vi "Run Auto Score.vi"(11 "Zip":path) -> (3 "Result":T1)   [LabVIEW 2024, in "Word Search Scorer.lvlib"]
uses:
  Word Search Scorer.lvlib
  Scoring Result.ctl
  <vilib>/Utility/error.llb/DialogType.ctl
  Result.ctl
  b176729e-45e3-4042-bf0b-439ceafae7e1.vi
  10f0845f-5e3d-49fd-8ad4-61868670d3b0.vi
panel:
  out "#":i32
  out "Additional Runs":i32
  out "Initial Run Time":dbl format="%_6f"
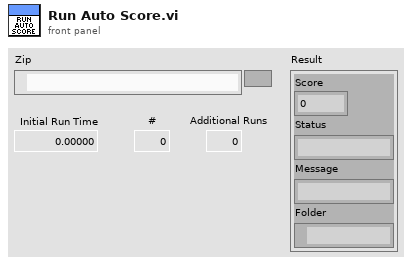
[diagram p1: front panel]
types:
  T1 = typedef "Word Search Scorer.lvlib/Scoring Result.ctl" = cluster{"Score":dbl, "Status":string, "Message":string, "Folder":path}
  T2 = typedef "DialogType.ctl" = u16
  T3 = typedef "Word Search Scorer.lvlib/Result.ctl" = enum16{"failed", "complete", "error", "timeout", "ineligible"}
  T4 = typedef "Word Search Scorer.lvlib/Solver VI Ref Type.ctl" = refnum<vi>
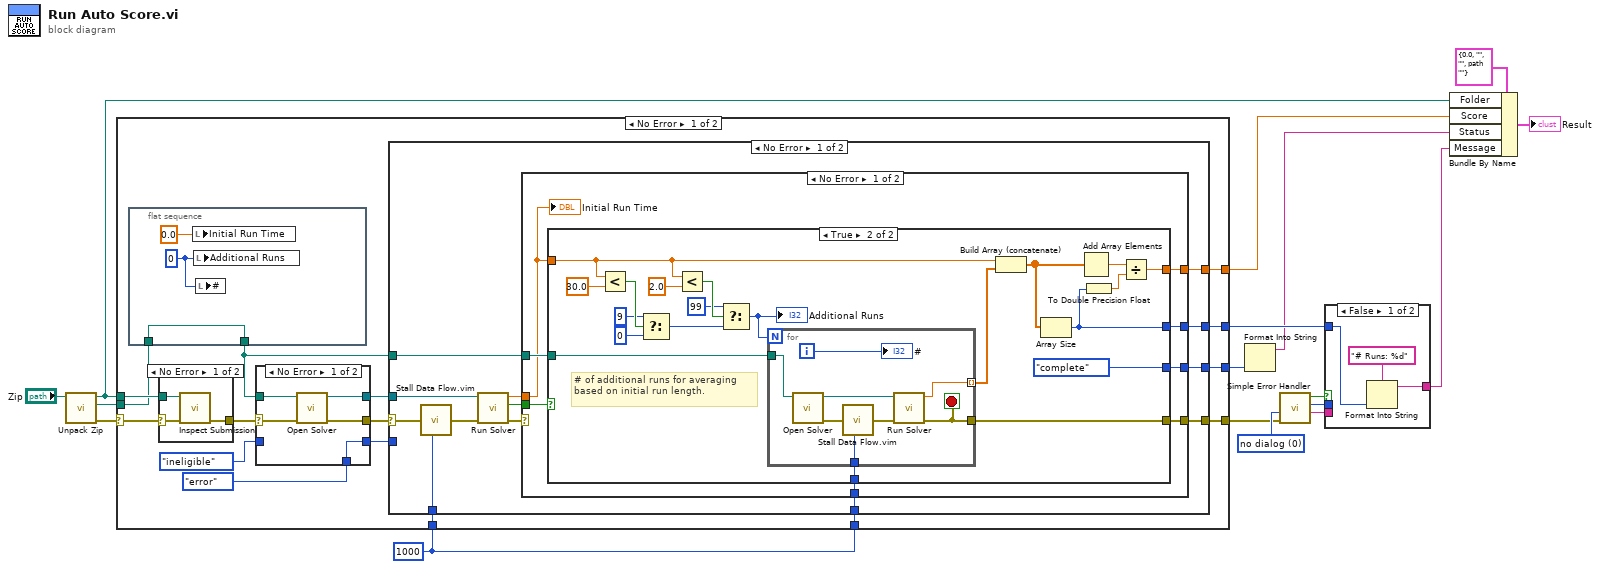
[diagram p0: block diagram]
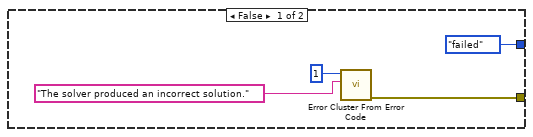
[diagram p2: hidden frame]
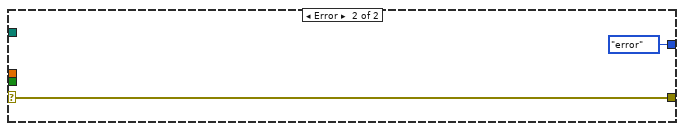
[diagram p3: hidden frame]
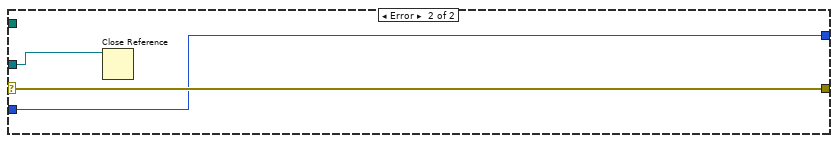
[diagram p4: hidden frame]
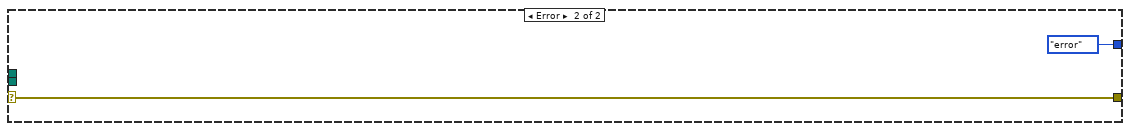
[diagram p7: hidden frame]
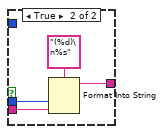
[diagram p8: hidden frame]
diagram:
  w1 = u32 1000 ("milliseconds to wait")
  w9 = T2 0 items=["no dialog", "OK message", "continue or stop message", "OK message + warnings", "continue/stop + warnings"] ("type of dialog (OK msg:1)")
  n1 = call "Unpack Zip.vi"("Zip"="Zip") -> ("error out"=w16:errorcluster, "Solver VI"=w13:path, "Folder"=w4:path)  [unwired: 8 in]
  n2 = case shown="No Error" w16 {
    selector: w16 -> [w33 w106]
    tunnel: w4 -> [w29 _]
    tunnel: w13 -> [w20 _]
    tunnel: [w25 Result."error" ("Result")] -> w8
    tunnel: [w24 w106] -> w7
    tunnel: [w23 _] -> w6
    tunnel: [w22 _] -> w5
    tunnel: w1 -> [w19 _]
    tunnel: w1 -> [w18 _]
    frame No Error {
      n3 = flat-sequence {
        tunnel: [w36] -> w21
        tunnel: w20 -> [w36]
        frame #0 {
          w34 = 0 ("Additional Runs")
          n4 = local write "Initial Run Time"(0.0 ("Initial Run Time")) -> ()
          n5 = local write "Additional Runs"(w34) -> ()
          n6 = local write "#"(w34) -> ()
        }
      }
      n7 = case shown="No Error" w33 {
        selector: w33 -> [w103 w105]
        tunnel: w29 -> [w104 _]
        tunnel: [w102 w105] -> w32
        frame No Error {
          n8 = call "Inspect Submission.vi"("error in (no error)"=w103, "Folder"=w104) -> ("error out"=w102:errorcluster)  [unwired: 7 in, 2 out]
        }
        frame Error {
        }
      }
      n9 = case shown="No Error" w32 {
        selector: w32 -> [w98 w101]
        tunnel: w21 -> [w99 _]
        tunnel: [w97 _] -> w30
        tunnel: [w96 w101] -> w31
        tunnel: [w95 w100] -> w27
        tunnel: Result."error" ("Result") -> [w95 _]
        tunnel: Result."ineligible" ("Result") -> [_ w100]
        frame No Error {
          n10 = call "Open Solver.vi"("error in (no error)"=w98, "Solver Path"=w99) -> ("error IO"=w96:errorcluster, "Solver VI"=w97:T4)  [unwired: 8 in]
        }
        frame Error {
        }
      }
      n11 = case shown="No Error" w31 {
        selector: w31 -> [w48 w94]
        tunnel: w30 -> [w49 w93]
        tunnel: [w43 w94] -> w24
        tunnel: w21 -> [w44 _]
        tunnel: [w42 _] -> w22
        tunnel: [w41 w92] -> w25
        tunnel: [w40 _] -> w23
        tunnel: w27 -> [_ w92]
        tunnel: w19 -> [w38 _]
        tunnel: w18 -> [w37 _]
        frame No Error {
          n12 = call "Stall Data Flow.vim"("value in"=w48, "milliseconds to wait"=w38) -> ("value out"=w39:errorcluster)  [unwired: 1 out]
          n13 = call "Run Solver.vi"("error in (no error)"=w39, "Solver VI"=w49) -> ("error out"=w47:errorcluster, "Completed"=w46:bool, "Run Time"=w45:dbl)  [unwired: 7 in]
          n14 = case shown="No Error" w47 {
            selector: w47 -> [_ w91]
            tunnel: w46 -> [w57 _]
            tunnel: w45 -> [w51 _]
            tunnel: w44 -> [w56 _]
            tunnel: [w55 w91] -> w43
            tunnel: [w54 _] -> w42
            tunnel: [w53 Result."error" ("Result")] -> w41
            tunnel: [w52 _] -> w40
            tunnel: w37 -> [w50 _]
            frame No Error {
              n15 = case shown="True" w57 {
                tunnel: w51 -> [_ w71]
                tunnel: w56 -> [_ w73]
                tunnel: [w60 w72] -> w55
                tunnel: [_ w66] -> w54
                tunnel: [Result."failed" ("Result") Result."complete" ("Result")] -> w53
                tunnel: [_ w64] -> w52
                tunnel: w50 -> [_ w62]
                frame False {
                  n16 = call <vilib>:"Error Cluster From Error Code.vi"("error message (\"\")"="The solver produced an incorrect solution.", "error code (0)"=1) -> ("error out"=w60:errorcluster)  [unwired: 7 in]
                }
                frame True {
                  # "# of additional runs for averaging based on initial run length."
                  n17 = Less?(x=w71, y=30.0) -> (x < y?=w80:bool)
                  n18 = Select(t=9, s=w80, f=0) -> (s? t:f=w76:i32)
                  n19 = Less?(x=w71, y=2.0) -> (x < y?=w75:bool)
                  n20 = Select(t=99, s=w75, f=w76) -> (s? t:f=w63:i32)
                  "Additional Runs" <- w63
                  n21 = for {
                    N: w63 -> [_]
                    tunnel: w73 -> [w87]
                    tunnel: [w86] -> w72
                    tunnel: [w85] -> w70 mode=indexing
                    tunnel: w62 -> [w82]
                    i -> [w84]
                    stop <- w86 stop-if-true
                    n22 = call "Open Solver.vi"("Solver Path"=w87) -> ("error IO"=w88:errorcluster, "Solver VI"=w89:T4)  [unwired: 9 in]
                    n23 = call "Stall Data Flow.vim"("value in"=w88, "milliseconds to wait"=w82) -> ("value out"=w83:errorcluster)  [unwired: 1 out]
                    n24 = call "Run Solver.vi"("error in (no error)"=w83, "Solver VI"=w89) -> ("error out"=w86:errorcluster, "Run Time"=w85:dbl)  [unwired: 7 in, 1 out]
                    "#" <- w84
                  }
                  n25 = Build Array (concatenate)(w71, w70) -> (w69:dbl[])
                  n26 = Array Size(array=w69) -> (size(s)=w64:i32)
                  n27 = Add Array Elements(numeric array=w69) -> (sum=w68:dbl)
                  n28 = To Double Precision Float(number=w64) -> (double precision float=w67:dbl)
                  n29 = Divide(x=w68, y=w67) -> (x/y=w66:dbl)
                }
              }
              "Initial Run Time" <- w51
            }
            frame Error {
            }
          }
        }
        frame Error {
          n30 = Close Reference(reference=w93) -> ()  [unwired: 1 in, 1 out]
        }
      }
    }
    frame Error {
    }
  }
  n31 = Format Into String(w8) -> (resulting string=w3:string)  [unwired: 3 in, 1 out]
  n32 = call <vilib>:"Simple Error Handler.vi"("type of dialog (OK msg:1)"=w9, "error in (no error)"=w7) -> ("error?"=w12:bool, "code out"=w11:i32, "source out"=w10:string)  [unwired: 3 in, 2 out]
  n33 = case shown="False" w12 {
    tunnel: w10 -> [_ w112]
    tunnel: w11 -> [_ w113]
    tunnel: w6 -> [w110 _]
    tunnel: [w108 w111] -> w2
    frame False {
      n34 = Format Into String(format string="# Runs: %d", w110) -> (resulting string=w108:string)  [unwired: 2 in, 1 out]
    }
    frame True {
      n35 = Format Into String(format string="(%d)\n%s", w113, w112) -> (resulting string=w111:string)  [unwired: 2 in, 1 out]
    }
  }
  n36 = Bundle By Name(cluster=T1 {"Score"=0.0, "Status"="", "Message"="", "Folder"=path ""} ("Scoring Result"), "Folder"=w4, "Score"=w5, "Status"=w3, "Message"=w2) -> (→"Result":T1)
